vi "SCCSup_Dynam GenErrorHandler.vi"(8 "error in (no error)":errorcluster, 10 "type of dialog (OK msg:1)":T1=1 items=["no dialog", "OK message", "continue or stop message", "OK message + warnings", "continue/stop + warnings"]) -> (0 "error out":errorcluster, 2 "message":string)   [LabVIEW 2017]
uses:
  <vilib>/Utility/error.llb/DialogType.ctl
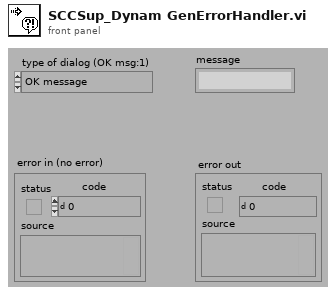
[diagram p1: front panel]
types:
  T1 = typedef "DialogType.ctl" = u16
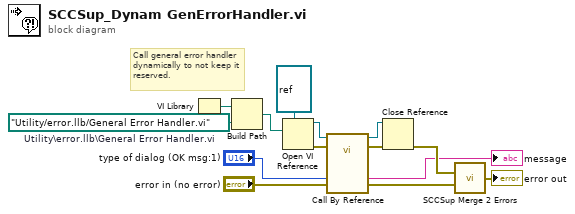
[diagram p0: block diagram]
diagram:
  w13 = path "Utility/error.llb/General Error Handler.vi"  # Utility\error.llb\General Error Handler.vi
  # "Call general error handler dynamically to not keep it reserved."
  n1 = VI Library() -> (path=w14:path)
  n2 = Build Path(base path=w14, name or relative path=w13) -> (appended path=w12:path)
  n3 = Open VI Reference(type specifier VI Refnum (for type only)=refnum<vi> refnum, vi path=w12) -> (vi reference=w8:refnum<vi>, error out=w9:errorcluster)  [unwired: 4 in]
  n4 = call-by-ref "?"(reference=w8, error in=w9, "type of dialog (OK msg:1)"="type of dialog (OK msg:1)", "error in (no error)"="error in (no error)") -> (reference out=w10:refnum<vi>, error out=w11:errorcluster, "message"=→"message":string, 15:"error out"=w5:errorcluster)  [unwired: 9 in, 3 out]
  n5 = Close Reference(reference=w10, error in (no error)=w11) -> (error out=w6:errorcluster)
  n6 = call <vilib>:"SCCSup Merge 2 Errors.vi"("Error IO 1"=w6, "Error IO 2"=w5) -> ("Error IO out"=→"error out":errorcluster)  [unwired: 13 in]
